vi "Analyze.vi"(0 "Analyze Distanz in":refnum<class "Analyze BeamDeviation.lvclass">, 1 "Create Overlay?":bool, 5 "Image in":T1, 7 "Parameters":variant, 9 "Results in":variant, 11 "error in (no error)":errorcluster) -> (4 "Analyze Distanz out":refnum<class "Analyze BeamDeviation.lvclass">, 6 "Image out":T1, 8 "Parameters out":variant, 10 "Results":variant, 15 "error out":errorcluster)   [LabVIEW 2014, in "Analyze.lvlib" / "Analyze BeamDeviation.lvclass"]
uses:
  Analyze BeamDeviation.lvclass
  <vilib>/vision/Image Controls.llb/IMAQ Image.ctl
  Analyze BaseClass/Analyze BaseClass.lvclass
  <vilib>/vision/NI_Vision_Development_Module.lvlib
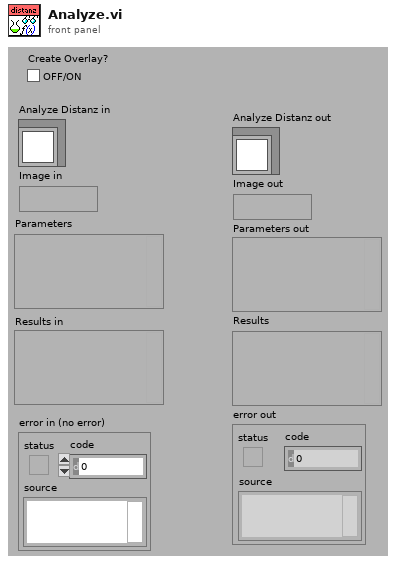
[diagram p1: front panel]
types:
  T1 = typedef "IMAQ Image.ctl" = refnum<image>
  T2 = typedef "ROI Descriptor" = cluster{"Global Rectangle":i32[], "Contours":cluster{"ID":enum32{"External", "Internal"}, "Type":u32, "Coordinates":i32[]}[]}
  T3 = cluster{"Desired Font (Application)":enum16{"User-specified Font", "Application Font", "System Font", "Dialog Font"}, "[User-specified Font]":cluster{"Font Name":string, "Size":i16, "Strikeout?":bool, "Italic?":bool, "Underline?":bool, "Outline?":bool, "Shadow?":bool, "Bold?":bool, "Rotation Angle":dbl}, "Horizontal Alignment":i16, "Vertical Alignment":i16}
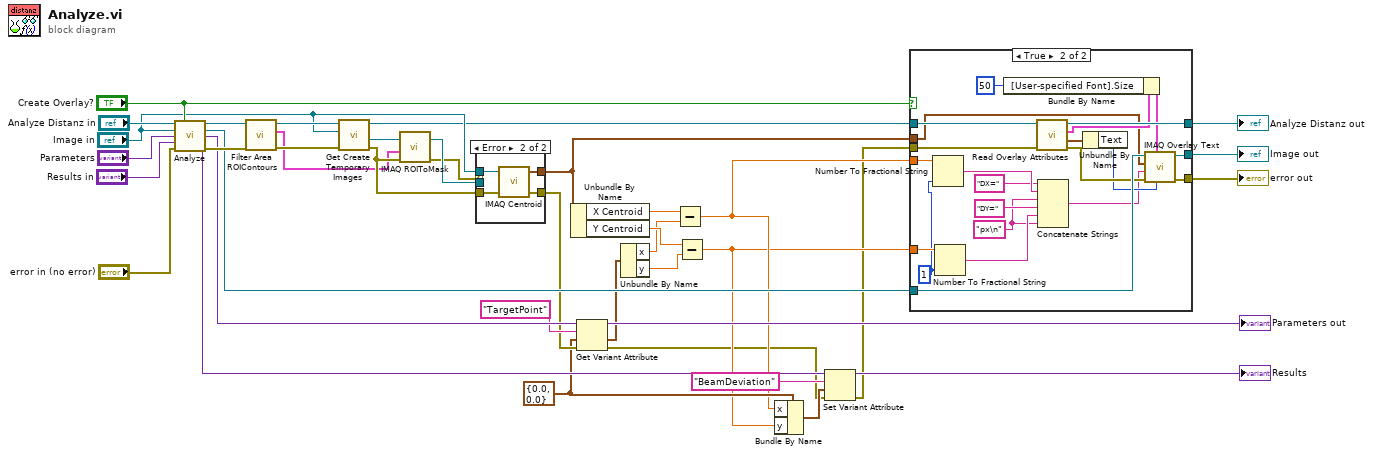
[diagram p0: block diagram]
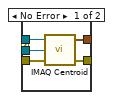
[diagram p2: hidden frame]
diagram:
  w11 = cluster{"x":dbl, "y":dbl} {"x"=0.0, "y"=0.0} ("point")
  n1 = call-parent "Analyze.vi"("Analyze BaseClass in"="Analyze Distanz in", "Create Overlay?"="Create Overlay?", "Image in"="Image in", "Parameters"="Parameters", "Results in"="Results in", "error in (no error)"="error in (no error)") -> ("Analyze BaseClass out"=w1:refnum<class "Analyze BeamDeviation.lvclass">, "Image out"=w32:T1, "Parameters out"=w26:variant, "Results"=w13:variant, "error out"=w35:errorcluster)  [unwired: 5 in]
  n2 = call-dynamic "Filter Area ROIContours.vi"("error in (no error)"=w35, "Analyze BaseClass in"=w1) -> ("error out"=w28:errorcluster, "ROI of Area type"=w2:T2, "Analyze BaseClass out"=w29:refnum<class "Analyze BeamDeviation.lvclass">)  [unwired: 7 in]
  n3 = call-dynamic "Get Create Temporary Images.vi"("error in (no error)"=w28, "Image in"="Image in", "Analyze BaseClass in"=w29) -> ("error out"=w4:errorcluster, "image mask"=w27:T1, "Analyze BaseClass out"=w20:refnum<class "Analyze BeamDeviation.lvclass">)  [unwired: 4 in, 2 out]
  n4 = call "IMAQ ROIToMask"("error in (no error)"=w4, "ROI Descriptor"=w2, "Image"=w27) -> ("error out"=w3:errorcluster, "Image Out"=w22:T1)  [unwired: 3 in, 1 out]
  n5 = case shown="Error" w3 {
    tunnel: "Image in" -> [w44 w48]
    tunnel: w22 -> [w43 _]
    tunnel: [w42 w47] -> w21
    tunnel: [w41 w46] -> w19
    tunnel: w4 -> [w40 w45]
    frame No Error {
      n6 = call "IMAQ Centroid"("error in (no error)"=w40, "Image Mask"=w43, "Image"=w44) -> ("error out"=w42:errorcluster, "Centroid"=w41:cluster{"X Centroid":sgl, "Y Centroid":sgl})  [unwired: 1 in]
    }
    frame Error {
      n7 = call "IMAQ Centroid"("error in (no error)"=w45, "Image"=w48) -> ("error out"=w47:errorcluster, "Centroid"=w46:cluster{"X Centroid":sgl, "Y Centroid":sgl})  [unwired: 2 in]
    }
  }
  n8 = Unbundle By Name(w19) -> ("X Centroid"=w18:sgl, "Y Centroid"=w16:sgl)
  n9 = Get Variant Attribute(Variant=w26, name="TargetPoint", default value (empty Variant)=w11, error in=w21) -> (duplicate Variant=→"Parameters out":variant, value=w17:cluster{"x":dbl, "y":dbl}, error out=w6:errorcluster)  [unwired: 1 out]
  n10 = Unbundle By Name(w17) -> ("x"=w15:dbl, "y"=w14:dbl)
  n11 = Subtract(x=w18, y=w15) -> (x-y=w10:dbl)
  n12 = Subtract(x=w16, y=w14) -> (x-y=w9:dbl)
  n13 = Bundle By Name(cluster=w11, "x"=w10, "y"=w9) -> (w8:cluster{"x":dbl, "y":dbl})
  n14 = Set Variant Attribute(Variant=w13, name="BeamDeviation", value=w8, error in=w6) -> (Variant out=→"Results":variant, error out=w5:errorcluster)  [unwired: 1 out]
  n15 = case shown="True" "Create Overlay?" {
    tunnel: w20 -> [w51 w73]
    tunnel: [w51 w72] -> w33
    tunnel: w32 -> [w50 w71]
    tunnel: [w50 w69] -> w30
    tunnel: [w49 w67] -> w31
    tunnel: w5 -> [w49 w66]
    tunnel: w19 -> [_ w63]
    tunnel: w10 -> [_ w62]
    tunnel: w9 -> [_ w61]
    frame False {
    }
    frame True {
      w55 = "px\n" ("string")
      w52 = i16 1 ("precision (6)")
      n16 = Number To Fractional String(number=w62, precision (6)=w52) -> (F-format string=w59:string)  [unwired: 2 in]
      n17 = Number To Fractional String(number=w61, precision (6)=w52) -> (F-format string=w60:string)  [unwired: 2 in]
      n18 = call-dynamic "Read Overlay Attributes.vi"("error in (no error)"=w66, "Analyze BaseClass in"=w73) -> ("error out"=w68:errorcluster, "Overlay colors"=w65:cluster{"Border":u32, "Text":u32}, "Font, Size & Style"=w70:T3, "Analyze BaseClass out"=w72:refnum<class "Analyze BeamDeviation.lvclass">)  [unwired: 5 in, 1 out]
      n19 = Bundle By Name(cluster=w70, "[User-specified Font].Size"=i16 50) -> (w54:T3)
      n20 = Concatenate Strings("DX=" ("string"), w59, w55, "DY=" ("string"), w60, w55) -> (w56:string)
      n21 = Unbundle By Name(w65) -> ("Text"=w64:u32)
      n22 = call "IMAQ Overlay Text"("Text Color (black)"=w64, "Font, Size & Style"=w54, "error in (no error)"=w68, "String"=w56, "Origin"=w63, "Image"=w71) -> ("error out"=w67:errorcluster, "Image Out"=w69:T1)  [unwired: 4 in]
    }
  }
  "error out" <- w31
  "Analyze Distanz out" <- w33
  "Image out" <- w30
